vi "Open File.vi"(7 "Readonly":bool, 8 "error in (no error)":errorcluster, 9 "File Path Control":path, 11 "Application refnum":refnum<k7>) -> (0 "error out":errorcluster, 2 "Presentation refnum out":refnum<k7>, 3 "Application refnum out":refnum<k7>)   [LabVIEW 2020, in "lvpptx.lvlib"]
uses:
  lvpptx.lvlib
panel:
  # "If the file is not found, \"not a refnum\"\nis returned as Presentation refnum out"
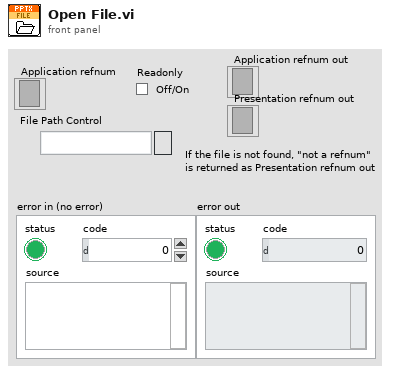
[diagram p1: front panel]
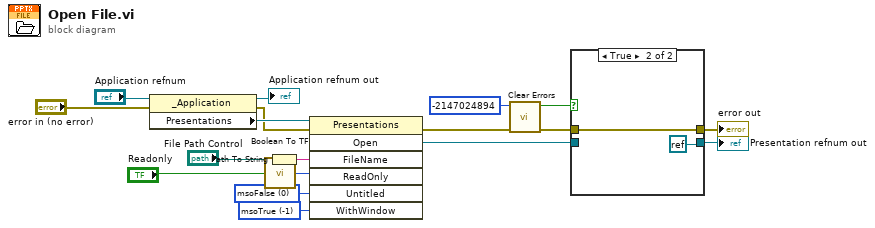
[diagram p0: block diagram]
diagram:
  w11 = 0 items=["msoTrue"=-1, "msoFalse"=0, "msoCTrue"=1, "msoTriStateToggle"=-3, "msoTriStateMixed"=-2] ("Untitled")
  w16 = -1 items=["msoTrue"=-1, "msoFalse"=0, "msoCTrue"=1, "msoTriStateToggle"=-3, "msoTriStateMixed"=-2] ("WithWindow")
  n1 = property class="_Application"(reference="Application refnum", error in="error in (no error)") -> (reference out=→"Application refnum out":refnum<k7>, error out=w15:errorcluster, "Presentations"=w17:refnum<k7>)
  n2 = call "Boolean To TF.vi"("Boolean"="Readonly") -> ("mso bool"=w10:i32)  [unwired: 4 in]
  n3 = Path To String(path="File Path Control") -> (string=w13:string)
  n4 = invoke class="Presentations" method="Open"(reference=w17, error in=w15, "FileName"=w13, "ReadOnly"=w10, "Untitled"=w11, "WithWindow"=w16) -> (error out=w7:errorcluster, "Open"=w3:refnum<k7>)  [unwired: 1 in, 5 out]
  n5 = call <vilib>:"Clear Errors.vi"("error in (no error)"=w7, "specific error code to clear (0: all)"=-2147024894) -> ("error out"=w4:errorcluster, "specific error cleared?"=w5:bool)  [unwired: 4 in]
  n6 = case shown="True" w5 {
    tunnel: w4 -> [w19 w21]
    tunnel: w3 -> [w20 _]
    tunnel: [w20 refnum<k0> refnum] -> w2
    tunnel: [w19 w21] -> w1
    frame False {
    }
    frame True {
    }
  }
  "error out" <- w1
  "Presentation refnum out" <- w2
